vi "savefile v1.1.vi"(0 "Length of array":i32, 2 "voltage":dbl[](array[numeric]), 4 "current":dbl[](array[numeric]), 6 "J":dbl[](array[numeric]), 7 "path of file":string, 10 "Voc":dbl, 11 "Power convertion efficiency":dbl, 14 "Jsc":dbl, 15 "current density":dbl[](array[numeric]), 18 "FF":dbl, 19 "Lamp Power":dbl) -> (20 "path":path, 23 "x = y?":bool)   [LabVIEW 2014]
panel:
  out "concatenated string":string
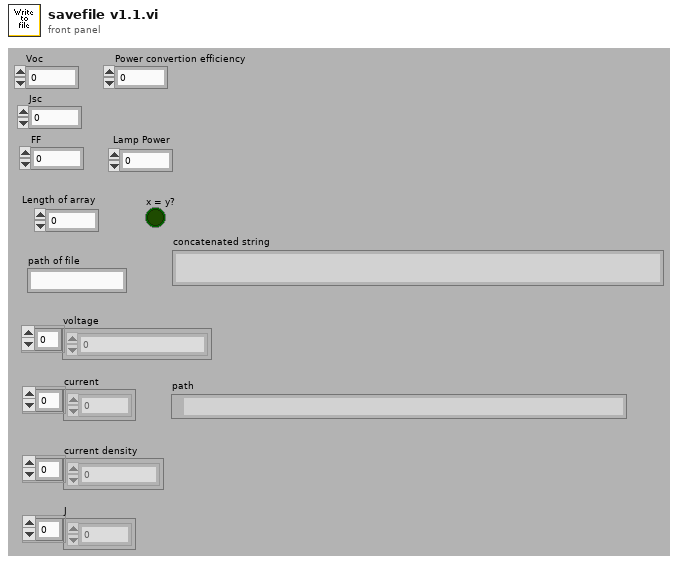
[diagram p1: front panel]
types:
  T1 = enum16{"open", "replace", "create", "open or create", "replace or create", "replace or create with confirmation"}
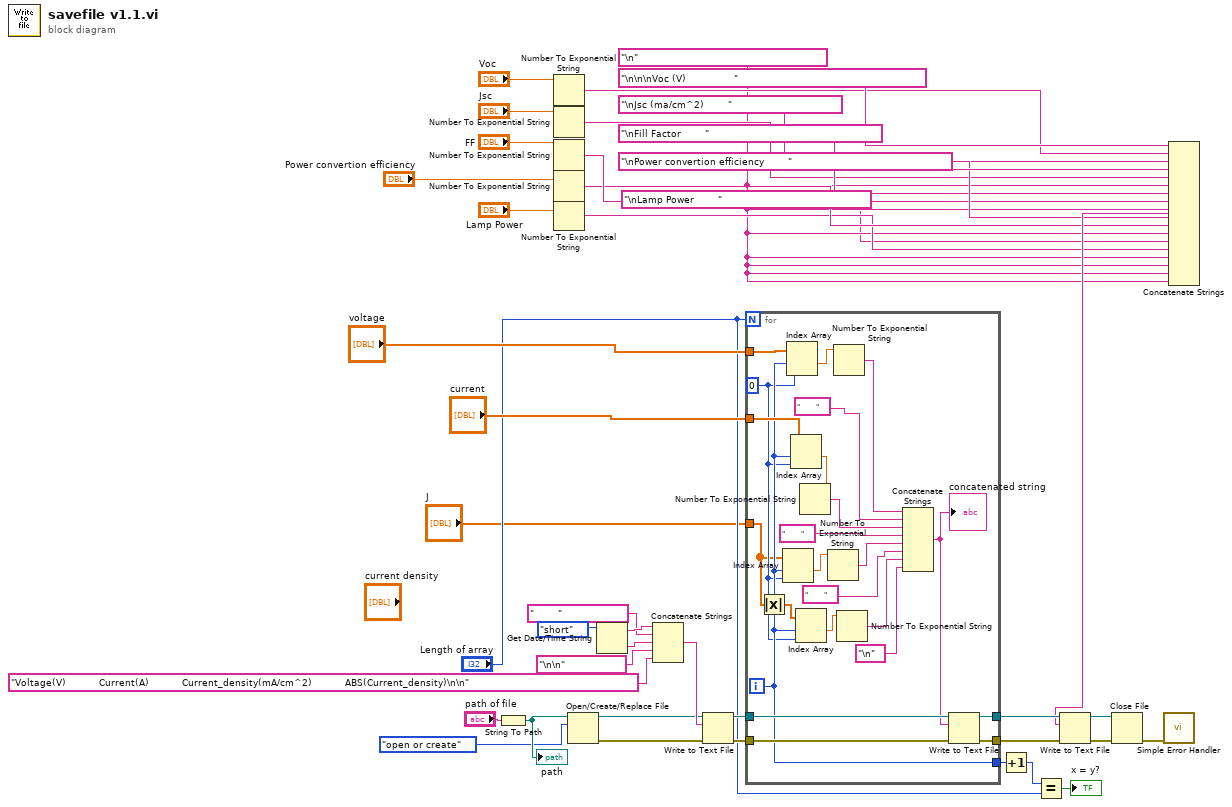
[diagram p0: block diagram]
diagram:
  w4 = "\n" ("string")
  n1 = String To Path(string="path of file") -> (path=w35:path)
  "path" <- w35
  n2 = Number To Exponential String(number="Voc") -> (E-format string=w14:string)  [unwired: 3 out]
  n3 = Number To Exponential String(number="Jsc") -> (E-format string=w13:string)  [unwired: 3 out]
  n4 = Number To Exponential String(number="FF") -> (E-format string=w12:string)  [unwired: 3 out]
  n5 = Number To Exponential String(number="Power convertion efficiency") -> (E-format string=w11:string)  [unwired: 3 out]
  n6 = Number To Exponential String(number="Lamp Power") -> (E-format string=w5:string)  [unwired: 3 out]
  n7 = Open/Create/Replace File(file path (use dialog)=w35, operation (0:open)=T1."open or create") -> (refnum out=w34:refnum<file>, error out=w33:errorcluster)  [unwired: 1 in, 4 out]
  n8 = Get Date/Time String(date format (0)=enum16{"short", "long", "abbreviated"}."short") -> (date string=w39:string, time string=w37:string)  [unwired: 2 out]
  n9 = Concatenate Strings(w39, "        " ("string"), w37, "\n\n" ("string"), "Voltage(V)           Current(A)           Current_density(mA/cm^2)           ABS(Current_density)\n\n" ("string")) -> (w36:string)
  n10 = Write to Text File(file (use dialog)=w34, text=w36, error in=w33) -> (refnum out=w42:refnum<file>, error out=w41:errorcluster)  [unwired: 2 out]
  n11 = for {
    N: "Length of array" -> [_]
    tunnel: [w66] -> w23
    tunnel: [w65] -> w22
    tunnel: w42 -> [w64]
    tunnel: w41 -> [w63]
    tunnel: "voltage" -> [w61]
    tunnel: "current" -> [w58]
    tunnel: [w52] -> w27
    tunnel: "J" -> [w45]
    i -> [w52]
    w51 = 0
    n12 = Absolute Value(x=w45) -> (abs(x)=w44:dbl[])
    n13 = Index Array(array=w45, index #1=w52, index #2=w51) -> (element #1=w50:dbl)  [unwired: 1 out]
    n14 = Index Array(array=w61, index #1=w52, index #2=w51) -> (element #1=w59:dbl)  [unwired: 1 out]
    n15 = Index Array(array=w58, index #1=w52, index #2=w51) -> (element #1=w60:dbl)  [unwired: 1 out]
    n16 = Index Array(array=w44, index #1=w52, index #2=w51) -> (element #1=w56:dbl)  [unwired: 1 out]
    n17 = Number To Exponential String(number=w60) -> (E-format string=w53:string)  [unwired: 3 out]
    n18 = Number To Exponential String(number=w50) -> (E-format string=w49:string)  [unwired: 3 out]
    n19 = Number To Exponential String(number=w59) -> (E-format string=w54:string)  [unwired: 3 out]
    n20 = Number To Exponential String(number=w56) -> (E-format string=w55:string)  [unwired: 3 out]
    n21 = Concatenate Strings(w54, "        " ("string"), w53, "        " ("string"), w49, "        " ("string"), w55, "\n" ("string")) -> (w62:string)
    "concatenated string" <- w62
    n22 = Write to Text File(file (use dialog)=w64, text=w62, error in=w63) -> (refnum out=w66:refnum<file>, error out=w65:errorcluster)  [unwired: 1 in, 1 out]
  }
  n23 = Increment(x=w27) -> (x+1=w26:i32)
  n24 = Equal?(x=w26, y="Length of array") -> (x = y?=→"x = y?":bool)
  n25 = Concatenate Strings("\n\n\nVoc (V)                " ("string"), w14, w4, "\nJsc (ma/cm^2)        " ("string"), w13, w4, "\nFill Factor        " ("string"), w12, w4, "\nPower convertion efficiency        " ("string"), w11, w4, "\nLamp Power        " ("string"), w5, w4, w4, w4, w4) -> (w17:string)
  n26 = Write to Text File(file (use dialog)=w23, text=w17, error in=w22) -> (refnum out=w20:refnum<file>, error out=w21:errorcluster)  [unwired: 2 out]
  n27 = Close File(refnum=w20, error in=w21) -> (error out=w43:errorcluster)  [unwired: 1 out]
  n28 = call <vilib>:"Simple Error Handler.vi"("error in (no error)"=w43) -> ()  [unwired: 1 in, 8 out]
